vi "GetThermalImage.vi"() -> ()   [LabVIEW 2024]
uses:
  libirimager.dll
panel:
  out "flagState":T1(ring)
  out "tempBox":sgl
  out "tempFlag":sgl
  out "tempChip":sgl
  out "timestampMedia":i64
  out "timestamp":i64
  out "counterHW":u32
  out "counter":u32
  out "data":u16[](array[numeric])
  out "h":i32
  out "w":i32
  out "Function Return":i32
  in  "height":i32
  in  "width":i32
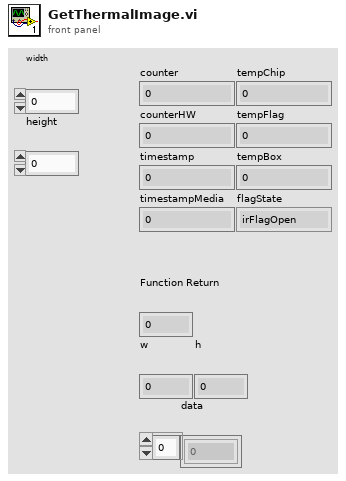
[diagram p1: front panel]
types:
  T1 = enum32{"irFlagOpen", "irFlagClose", "irFlagOpening", "irFlagClosing", "irFlagError"}
  T2 = cluster{"counter":u32, "counterHW":u32, "timestamp":i64, "timestampMedia":i64, "flagState":enum32{"irFlagOpen", "irFlagClose", "irFlagOpening", "irFlagClosing", "irFlagError"}, "tempChip":sgl, "tempFlag":sgl, "tempBox":sgl}
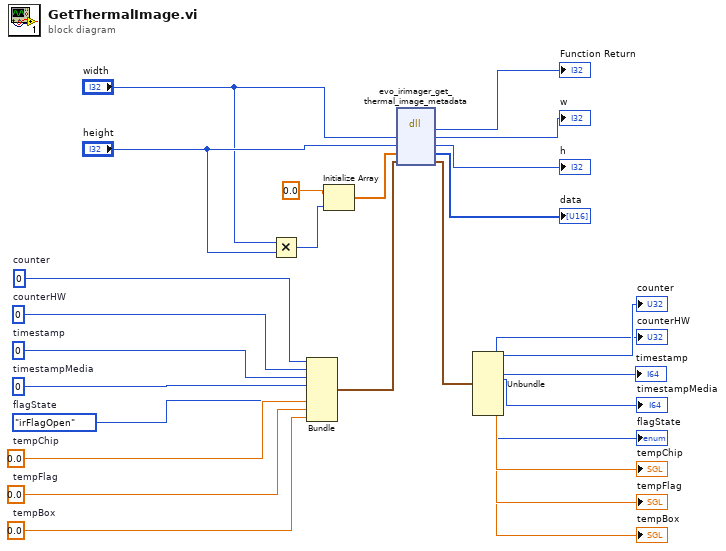
[diagram p0: block diagram]
diagram:
  w10 = T1."irFlagOpen"  # flagState
  w13 = sgl 0.0  # tempBox
  w14 = sgl 0.0  # tempFlag
  w15 = sgl 0.0  # tempChip
  w16 = i64 0  # timestampMedia
  w17 = i64 0  # timestamp
  w12 = u32 0  # counterHW
  w11 = u32 0  # counter
  n1 = Multiply(x="width", y="height") -> (x*y=w22:i32)
  n2 = Bundle("counter"=w11, "counterHW"=w12, "timestamp"=w17, "timestampMedia"=w16, "flagState"=w10, "tempChip"=w15, "tempFlag"=w14, "tempBox"=w13) -> (w9:T2)  [unwired: 1 in]
  n3 = Initialize Array(0.0 ("element"), w22) -> (w26:dbl[])
  n4 = dll-call lib="C:/Users/mayhe/OneDrive/Documents/GitHub/In-situ-monitoring-of-powder-bed-fusion-additive-manufacturing/system_development/Orichalcum/v0.2/Software_design/thermal-camera/libirimager.dll" fn="evo_irimager_get_thermal_image_metadata"("w"="width", "h"="height", "data"=w26, "metadata"=w9) -> ("Rückgabetyp"=→"Function Return":i32, "w"=→"w":i32, "h"=→"h":i32, "data"=→"data":u16[], "metadata"=w1:T2)  [unwired: 3 in, 2 out]
  n5 = Unbundle(w1) -> ("counter"=→"counter":u32, "counterHW"=→"counterHW" →"timestamp":u32, "timestampMedia"=→"timestampMedia":i64, "flagState"=→"flagState":T1, "tempChip"=→"tempChip":sgl, "tempFlag"=→"tempFlag":sgl, "tempBox"=→"tempBox":sgl)  [unwired: 1 out]
